vi "Util_TrajectoryState_Meters_To_Inches.vi"(11 "absTRAJECTORY":T1={"TimeSeconds"=0.0, "Velocity"=0.0, "Acceleration"=0.0, "POSE"={"TRANSLATION"={"X"=0.0, "Y"=0.0}, "ROTATION"={"VALUE"=0.0, "COS"=1.0, "SIN"=0.0}}, "Curvature"=0.0} {"POSE"."ROTATION"."SIN" format="%13.4f"; "POSE"."ROTATION"."COS" format="%13.4f"; "POSE"."ROTATION"."VALUE" format="%13.4f"; "POSE"."TRANSLATION"."Y" format="%14.3f"; "POSE"."TRANSLATION"."X" format="%14.3f"}) -> (3 "outputRelativeTRAJECTORY":T1={"TimeSeconds"=0.0, "Velocity"=0.0, "Acceleration"=0.0, "POSE"={"TRANSLATION"={"X"=0.0, "Y"=0.0}, "ROTATION"={"VALUE"=0.0, "COS"=1.0, "SIN"=0.0}}, "Curvature"=0.0} {"POSE"."ROTATION"."SIN" format="%13.4f"; "POSE"."ROTATION"."COS" format="%13.4f"; "POSE"."ROTATION"."VALUE" format="%13.4f"; "POSE"."TRANSLATION"."Y" format="%14.3f"; "POSE"."TRANSLATION"."X" format="%14.3f"})   [LabVIEW 2019, in "Trajectory_Library.lvlib"]
doc: "Utility function to convert a trajectory state from meters, radians to inches and degrees. This is for DISPLAY ONLY. Do not SAMPLE or perform other operations on this data!!!"
uses:
  Trajectory_Library.lvlib
  TypeDef/TRAJ_STATE.ctl
  TypeDef/POSE2D.ctl
  TypeDef/TRANSLATION2D.ctl
  TypeDef/ROTATION2D.ctl
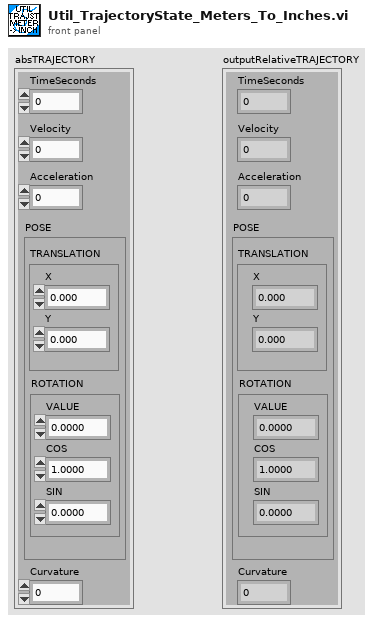
[diagram p1: front panel]
types:
  T1 = typedef "Trajectory_Library.lvlib/TRAJ_STATE.ctl" = cluster{"TimeSeconds":dbl, "Velocity":dbl, "Acceleration":dbl, "POSE":T2, "Curvature":dbl}
  T2 = typedef "Trajectory_Library.lvlib/POSE2D.ctl" = cluster{"TRANSLATION":T3, "ROTATION":T4}
  T3 = typedef "Trajectory_Library.lvlib/TRANSLATION2D.ctl" = cluster{"X":dbl, "Y":dbl}
  T4 = typedef "Trajectory_Library.lvlib/ROTATION2D.ctl" = cluster{"VALUE":dbl, "COS":dbl, "SIN":dbl}
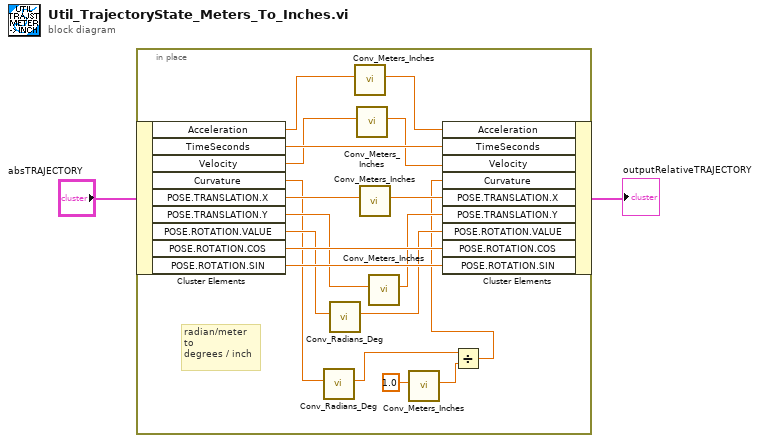
[diagram p0: block diagram]
diagram:
  n1 = in-place {
    # "radian/meter\nto\ndegrees / inch"
    n2 = in-place-cluster #1("absTRAJECTORY") -> ("Acceleration"=w10:dbl, "TimeSeconds"=w20:dbl, "Velocity"=w12:dbl, "Curvature"=w13:dbl, "POSE.TRANSLATION.X"=w15:dbl, "POSE.TRANSLATION.Y"=w16:dbl, "POSE.ROTATION.VALUE"=w17:dbl, "POSE.ROTATION.COS"=w19:dbl, "POSE.ROTATION.SIN"=w18:dbl)
    n3 = call "Conv_Radians_Deg.vi"("Radians"=w13) -> ("Degrees"=w4:dbl)  [unwired: 10 in]
    n4 = call "Conv_Radians_Deg.vi"("Radians"=w17) -> ("Degrees"=w8:dbl)  [unwired: 10 in]
    n5 = call "Conv_Meters_Inches.vi"("Meters"=w10) -> ("Inches"=w9:dbl)  [unwired: 10 in]
    n6 = call "Conv_Meters_Inches.vi"("Meters"=w12) -> ("Inches"=w11:dbl)  [unwired: 10 in]
    n7 = call "Conv_Meters_Inches.vi"("Meters"=w15) -> ("Inches"=w14:dbl)  [unwired: 10 in]
    n8 = call "Conv_Meters_Inches.vi"("Meters"=w16) -> ("Inches"=w7:dbl)  [unwired: 10 in]
    n9 = call "Conv_Meters_Inches.vi"("Meters"=1.0) -> ("Inches"=w5:dbl)  [unwired: 10 in]
    n10 = Divide(x=w4, y=w5) -> (x/y=w3:dbl)
    n11 = in-place-cluster #1("Acceleration"=w9, "TimeSeconds"=w20, "Velocity"=w11, "Curvature"=w3, "POSE.TRANSLATION.X"=w14, "POSE.TRANSLATION.Y"=w7, "POSE.ROTATION.VALUE"=w8, "POSE.ROTATION.COS"=w19, "POSE.ROTATION.SIN"=w18) -> (→"outputRelativeTRAJECTORY":T1)
  }
